vi "Write directory.vi"(8 "error in (no error)":errorcluster, 11 "Log File in":refnum<class "Log File.lvclass">) -> (0 "error out":errorcluster, 3 "Log File out":refnum<class "Log File.lvclass">)   [LabVIEW 2018, in "Log File.lvclass"]
uses:
  Log File.lvclass
  Log File.lvclass/Log File.ctl
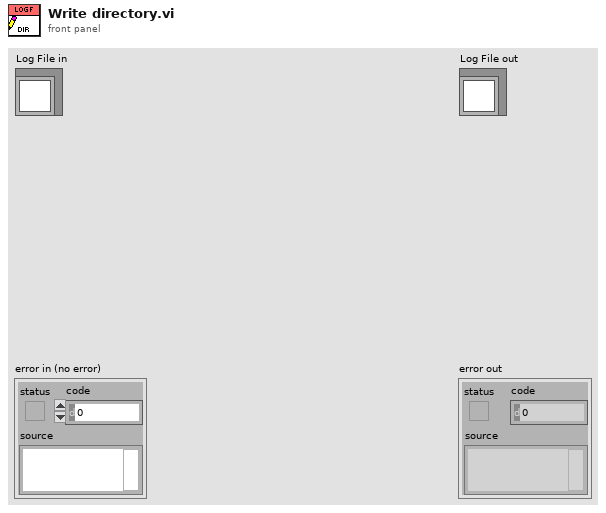
[diagram p1: front panel]
types:
  T1 = typedef "LVDateTimeRec.ctl" = cluster{"fractional second":dbl, "second":i32, "minute":i32, "hour":i32, "day of month":i32, "month":i32, "year":i32, "day of week":i32, "day of year":i32, "DST":i32}
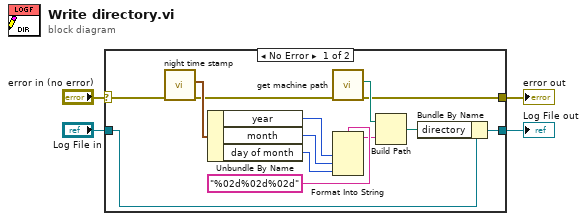
[diagram p0: block diagram]
diagram:
  n1 = case shown="No Error" "error in (no error)" {
    selector: "error in (no error)" -> [w7 w18]
    tunnel: [w5 w18] -> w3
    tunnel: [w10 w19] -> w1
    tunnel: "Log File in" -> [w11 w19]
    frame No Error {
      n2 = call "night time stamp.vi"("error in (no error)"=w7) -> ("error out"=w6:errorcluster, "date time rec"=w8:T1)  [unwired: 9 in]
      n3 = Unbundle By Name(w8) -> ("year"=w17:i32, "month"=w16:i32, "day of month"=w15:i32)
      n4 = call "get machine path.vi"("error in (no error) 2"=w6) -> ("error in (no error)"=w5:errorcluster, "machine path"=w9:path)  [unwired: 9 in]
      n5 = Format Into String(format string="%02d%02d%02d", w17, w16, w15) -> (resulting string=w13:string)  [unwired: 2 in, 1 out]
      n6 = Build Path(base path=w9, name or relative path=w13) -> (appended path=w12:path)
      n7 = Bundle By Name(cluster=w11, "directory"=w12) -> (w10:refnum<class "Log File.lvclass">)
    }
    frame Error {
    }
  }
  "error out" <- w3
  "Log File out" <- w1
